vi "Path.vi"(9 "error in (no error)":errorcluster, 10 "selected path":path) -> (0 "appended path":path, 1 "Exist?":bool, 2 "Boolean":bool, 3 "error out":errorcluster)   [LabVIEW 2013, in "Test_Libraries.lvlib"]
uses:
  Proyecto/Test_Libraries.lvlib
panel:
  out "Name":string
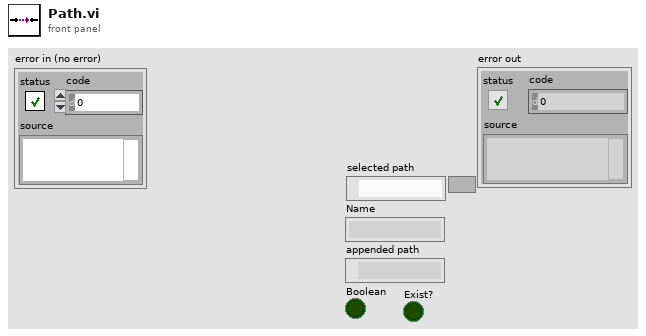
[diagram p1: front panel]
types:
  T1 = enum16{"open", "replace", "create", "open or create", "replace or create", "replace or create with confirmation"}
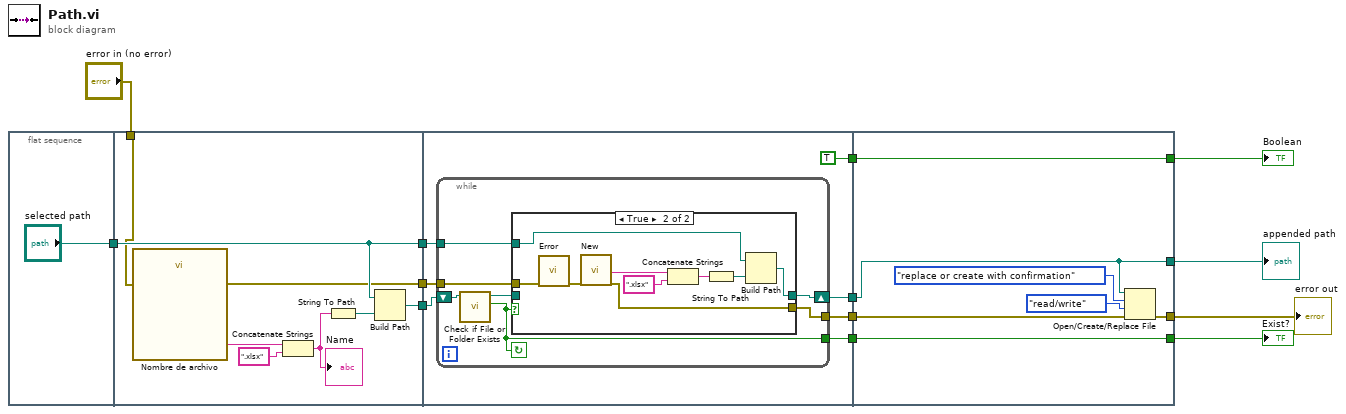
[diagram p0: block diagram]
diagram:
  n1 = flat-sequence {
    tunnel: ["selected path"] -> w13
    tunnel: w13 -> [w17]
    tunnel: [w18] -> w12
    tunnel: [w17] -> w11
    tunnel: [w16] -> w4
    tunnel: "error in (no error)" -> [w15]
    tunnel: w12 -> [w29]
    tunnel: w11 -> [w28]
    tunnel: [w27] -> w7
    tunnel: [TRUE] -> w6
    tunnel: [w25] -> w5
    tunnel: w4 -> [w24]
    tunnel: [w23] -> w3
    tunnel: [w53] -> w8
    tunnel: [w54] -> w9
    tunnel: [w52] -> w10
    tunnel: w7 -> [w52]
    tunnel: w6 -> [w54]
    tunnel: w5 -> [w53]
    tunnel: [w49] -> w2
    tunnel: w3 -> [w48]
    frame #0 {
    }
    frame #1 {
      n2 = call "Nombre de archivo"("error in (no error)"=w15) -> ("Nombre"=w22:string, "error out"=w16:errorcluster)  [unwired: 16 in, 1 out]
      n3 = Concatenate Strings(w22, ".xlsx" ("string")) -> (w19:string)
      "Name" <- w19
      n4 = String To Path(string=w19) -> (path=w20:path)
      n5 = Build Path(base path=w17, name or relative path=w20) -> (appended path=w18:path)
    }
    frame #2 {
      n6 = while {
        shift-right: [w34] -> w27
        shift-left: w29 -> [w36]
        tunnel: w28 -> [w35]
        tunnel: [w32] -> w25
        tunnel: w24 -> [w31]
        tunnel: [w30] -> w23
        stop <- w32 continue-if-true
        n7 = call <vilib>:"Check if File or Folder Exists.vi"("path"=w36) -> ("file or folder exists?"=w32:bool, "dup path"=w33:path)  [unwired: 8 in, 1 out]
        n8 = case shown="True" w32 {
          tunnel: w35 -> [_ w43]
          tunnel: [w38 w42] -> w34
          tunnel: w33 -> [w38 _]
          tunnel: w31 -> [w37 w40]
          tunnel: [w37 w39] -> w30
          frame False {
          }
          frame True {
            n9 = call "Error"("error in (no error)"=w40) -> ("error out"=w46:errorcluster)  [unwired: 9 in, 1 out]
            n10 = call "New"("error in (no error)"=w46) -> ("Nombre"=w41:string, "error out"=w39:errorcluster)  [unwired: 16 in, 1 out]
            n11 = Concatenate Strings(w41, ".xlsx" ("string")) -> (w47:string)
            n12 = String To Path(string=w47) -> (path=w44:path)
            n13 = Build Path(base path=w43, name or relative path=w44) -> (appended path=w42:path)
          }
        }
      }
    }
    frame #3 {
      n14 = Open/Create/Replace File(file path (use dialog)=w52, error in=w48, operation (0:open)=T1."replace or create with confirmation", access (0:read/write)=enum16{"read/write", "read-only", "write-only"}."read/write") -> (error out=w49:errorcluster)  [unwired: 2 in, 2 out]
    }
  }
  "appended path" <- w10
  "Boolean" <- w9
  "Exist?" <- w8
  "error out" <- w2
